vi "Spi Master 128-bit.vi"(0 "spi input":T1, 5 "manual assert chip select":bool, 7 "start strobe":bool, 9 "data to write":bool[](array[boolean]), 11 "MOSI output enable done":bool=TRUE, 13 "spi transfer settings":T2 {"Direction Change Bit" max=64 step=1; "Transfer Length (bits)" min=1 max=64 step=1}) -> (4 "spi output":T3, 8 "read data valid":bool, 10 "read data":bool[](array[boolean]), 14 "ready for input":bool)   [LabVIEW 2015, in "SPI API.lvlib"]
doc: "<b>This VI must be placed in a single-cycle timed loop for guaranteed behavior.</b>\n\nThis VI implements a SPI master that is compliant with both 4-wire (unidirectional input and output data) and 3-wire (bidirectional input/output data) SPI transfers. \n\nPlease see the documentation included with this example for details on how to include this VI into your application.\n\n\"Start strobe\" should be asserted only when \"data to write\" is valid. \"Data to write\" is latched when the start strobe asserts."
uses:
  <userlib>/_NI SPI IP/FPGA/Controllers/Public/Spi Master Outputs.ctl
  <userlib>/_NI SPI IP/FPGA/Controllers/Public/Transfer Settings.ctl
  <userlib>/_NI SPI IP/FPGA/Controllers/Public/Spi Master Inputs.ctl
  Controls/Controller Interface.ctl
  Controls/Master State.ctl
  SPI API.lvlib
  <userlib>/_NI SPI IP/FPGA/Controllers/NI SPI IP FPGA.lvlib
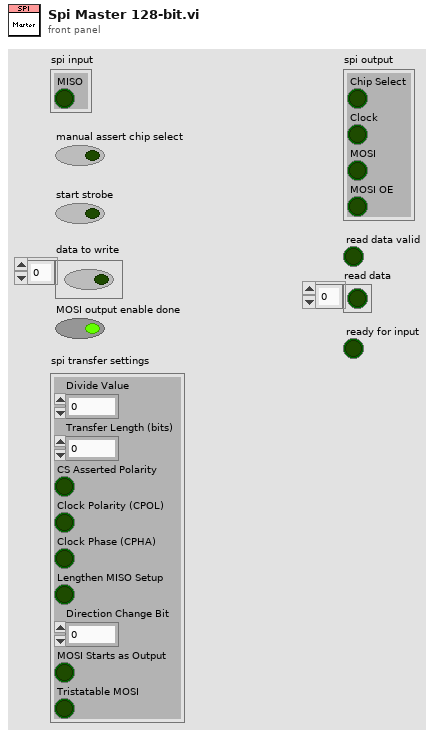
[diagram p1: front panel]
types:
  T1 = typedef "NI SPI IP FPGA.lvlib/Spi Master Inputs.ctl" = cluster{"MISO":bool}
  T2 = typedef "NI SPI IP FPGA.lvlib/Transfer Settings.ctl" = cluster{"Divide Value":u8, "Transfer Length (bits)":u8, "CS Asserted Polarity":bool, "Clock Polarity (CPOL)":bool, "Clock Phase (CPHA)":bool, "Lengthen MISO Setup":bool, "Direction Change Bit":u8, "MOSI Starts as Output":bool, "Tristatable MOSI":bool}
  T3 = typedef "NI SPI IP FPGA.lvlib/Spi Master Outputs.ctl" = cluster{"Chip Select":bool, "Clock":bool, "MOSI":bool, "MOSI OE":bool}
  T4 = typedef "SPI API.lvlib/Master State.ctl" = enum16{"Idle", "Load", "AssertChipSelect", "SendData", "DeassertChipSelect", "Done", "Change MOSI Direction", "WaitForDirChangeDone"}
  T5 = typedef "SPI API.lvlib/Controller Interface.ctl" = cluster{"Load":bool, "Divider Pulse":bool, "Enable Data":bool, "Clear Mosi":bool}
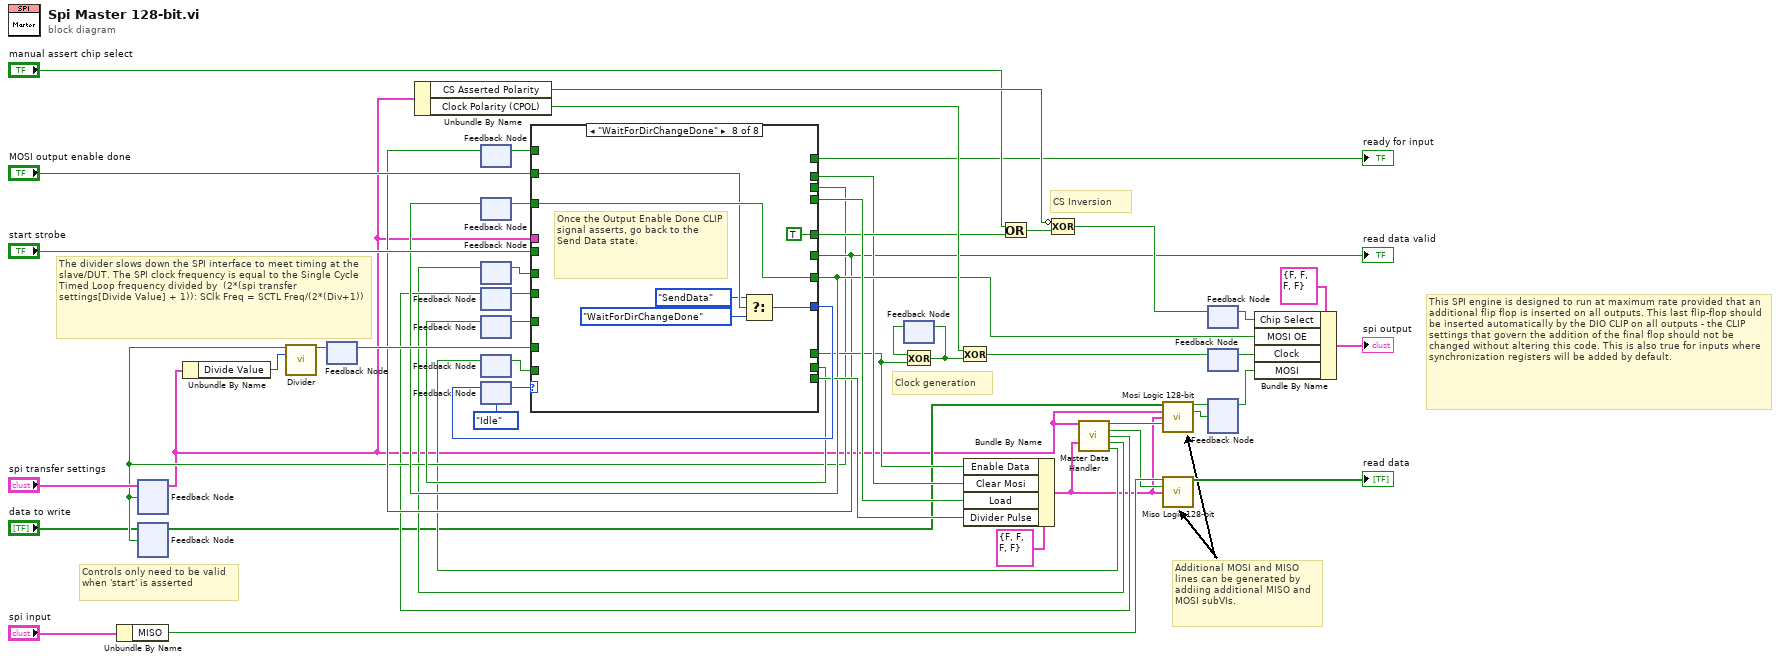
[diagram p0: block diagram]
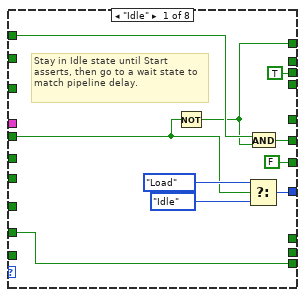
[diagram p2: hidden frame]
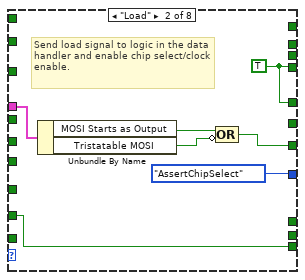
[diagram p3: hidden frame]
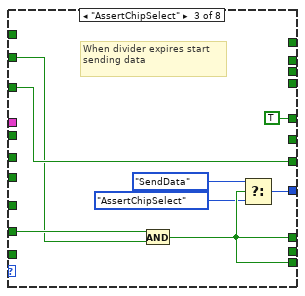
[diagram p4: hidden frame]
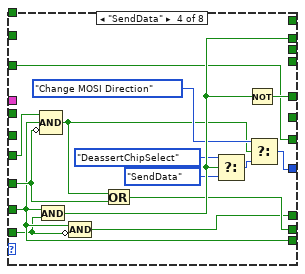
[diagram p5: hidden frame]
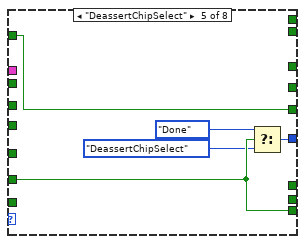
[diagram p6: hidden frame]
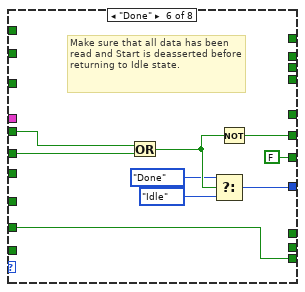
[diagram p7: hidden frame]
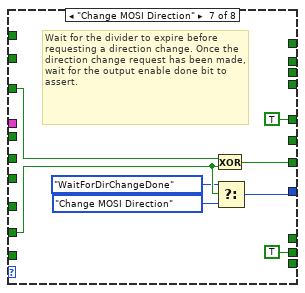
[diagram p8: hidden frame]
diagram:
  # "CS Inversion"
  # "Additional MOSI and MISO lines can be generated by addiing additional MISO and MOSI subVIs."
  # "Controls only need to be valid when 'start' is asserted"
  # "Clock generation"
  # "This SPI engine is designed to run at maximum rate provided that an additional flip flop is inserted on all outputs. This last flip-flop should be inserted automatically by the DIO CLIP on all outputs - the CLIP settings that govern the addition of the final flop should not be changed without altering this code. This is also true for inputs where synchronization registers will be added by default."
  # "The divider slows down the SPI interface to meet timing at the slave/DUT. The SPI clock frequency is equal to the Single Cycle Timed Loop frequency divided by  (2*(spi transfer settings[Divide Value] + 1)): SClk Freq = SCTL Freq/(2*(Div+1))"
  n1 = Unbundle By Name("spi input") -> ("MISO"=w4:bool)
  n2 = feedback #1() -> (w8:T2)  [unwired: 1 in]
  n3 = feedback #2() -> (w9:bool[])  [unwired: 1 in]
  n4 = Unbundle By Name(w8) -> ("Divide Value"=w15:u8)
  n5 = feedback #3() -> (w40:bool)  [unwired: 1 in]
  n6 = Unbundle By Name(w8) -> ("CS Asserted Polarity"=w37:bool, "Clock Polarity (CPOL)"=w49:bool)
  n7 = feedback #4() -> (w19:bool)  [unwired: 1 in]
  n8 = feedback #5() -> (w32:bool)  [unwired: 1 in]
  n9 = feedback #6() -> (w43:bool)  [unwired: 1 in]
  n10 = feedback #7() -> (w33:bool)  [unwired: 1 in]
  n11 = feedback #8() -> (w29:bool)  [unwired: 1 in]
  n12 = feedback #9() -> (w50:bool)  [unwired: 1 in]
  n13 = feedback #10(Master_State."Idle" ("state type")) -> (w52:T4)
  n14 = case shown="\"WaitForDirChangeDone\"" w52 {
    tunnel: [w63 Master_State."AssertChipSelect" ("state type") w78 w90 w98 w107 w114 w120] -> w53
    tunnel: w40 -> [w61 w69 w75 w87 w96 w104 w110 _]
    tunnel: [w58 _ _ _ _ _ _ _] -> w21
    tunnel: "start strobe" -> [w54 _ _ _ _ w106 _ _]
    tunnel: [_ w70 TRUE w93 _ _ TRUE ("Clock") TRUE ("Clock")] -> w36
    tunnel: w50 -> [_ _ _ w86 _ _ _ _]
    tunnel: [_ _ w73 w85 _ _ _ _] -> w22
    tunnel: [_ w70 _ _ _ _ _ _] -> w47
    tunnel: [TRUE ("Clock") _ _ _ _ _ _ _] -> w16
    tunnel: [_ _ _ w92 _ _ _ _] -> w23
    tunnel: w43 -> [_ _ _ _ _ w105 _ _]
    tunnel: w33 -> [_ _ _ w83 _ _ _ _]
    tunnel: [FALSE w65 w76 w84 w97 FALSE w111 w121] -> w24
    tunnel: w32 -> [_ _ w76 w84 w97 _ w112 w121]
    tunnel: [w61 w69 w73 w87 w96 w104 _ _] -> w31
    tunnel: [_ _ _ w88 _ _ TRUE _] -> w30
    tunnel: w29 -> [_ _ _ w89 _ _ _ _]
    tunnel: w8 -> [_ w68 _ _ _ _ _ _]
    tunnel: "MOSI output enable done" -> [_ _ w74 _ _ _ _ w118]
    tunnel: [w60 _ _ _ _ w102 _ _] -> w20
    tunnel: w19 -> [w59 _ _ _ _ _ _ _]
    frame "Idle" {
      # "Stay in Idle state until Start asserts, then go to a wait state to match pipeline delay."
      n15 = Not(x=w54) -> (.not. x?=w58:bool)
      n16 = Select(t=Master_State."Load" ("state type"), s=w54, f=Master_State."Idle" ("state type")) -> (s? t:f=w63:T4)
      n17 = And(x=w59, y=w58) -> (x .and. y?=w60:bool)
    }
    frame "Load" {
      w70 = TRUE ("Clock")
      # "Send load signal to logic in the data handler and enable chip select/clock enable."
      n18 = Unbundle By Name(w68) -> ("MOSI Starts as Output"=w67:bool, "Tristatable MOSI"=w66:bool)
      n19 = Compound Arithmetic op=OR(w67, invert w66) -> (w65:bool)
    }
    frame "AssertChipSelect" {
      # "When divider expires start sending data"
      n20 = And(x=w75, y=w74) -> (x .and. y?=w73:bool)
      n21 = Select(t=Master_State."SendData" ("state type"), s=w73, f=Master_State."AssertChipSelect" ("state type")) -> (s? t:f=w78:T4)
    }
    frame "SendData" {
      n22 = And(x=w87, y=w86) -> (x .and. y?=w92:bool)
      n23 = Compound Arithmetic op=AND(w83, w87, invert w89) -> (w81:bool)
      n24 = Compound Arithmetic op=AND(w87, invert w86) -> (w85:bool)
      n25 = Or(x=w81, y=w89) -> (x .or. y?=w88:bool)
      n26 = Select(t=Master_State."DeassertChipSelect" ("state type"), s=w92, f=Master_State."SendData" ("state type")) -> (s? t:f=w91:T4)
      n27 = Not(x=w92) -> (.not. x?=w93:bool)
      n28 = Select(t=Master_State."Change MOSI Direction" ("state type"), s=w81, f=w91) -> (s? t:f=w90:T4)
    }
    frame "DeassertChipSelect" {
      n29 = Select(t=Master_State."Done" ("state type"), s=w96, f=Master_State."DeassertChipSelect" ("state type")) -> (s? t:f=w98:T4)
    }
    frame "Done" {
      # "Make sure that all data has been read and Start is deasserted before returning to Idle state."
      n30 = Or(x=w106, y=w105) -> (x .or. y?=w103:bool)
      n31 = Select(t=Master_State."Done" ("state type"), s=w103, f=Master_State."Idle" ("state type")) -> (s? t:f=w107:T4)
      n32 = Not(x=w103) -> (.not. x?=w102:bool)
    }
    frame "Change MOSI Direction" {
      # "Wait for the divider to expire before requesting a direction change. Once the direction change request has been made, wait for the output enable done bit to assert."
      n33 = Exclusive Or(1:w110, 2:w112) -> (0:w111:bool)
      n34 = Select(t=Master_State."WaitForDirChangeDone" ("state type"), s=w110, f=Master_State."Change MOSI Direction" ("state type")) -> (s? t:f=w114:T4)
    }
    frame "WaitForDirChangeDone" {
      # "Once the Output Enable Done CLIP signal asserts, go back to the Send Data state."
      n35 = Select(t=Master_State."SendData" ("state type"), s=w118, f=Master_State."WaitForDirChangeDone" ("state type")) -> (s? t:f=w120:T4)
    }
  }
  "ready for input" <- w21
  "read data valid" <- w20
  n36 = feedback-in #1("spi transfer settings", w16) -> ()
  n37 = feedback-in #2("data to write", w16) -> ()
  n38 = call "Divider.vi"("reset"=w16, "divide value"=w15) -> ("count done"=w14:bool)  [unwired: 13 in]
  n39 = feedback-in #3(w14) -> ()
  n40 = feedback-in #4(w20) -> ()
  n41 = feedback-in #5(w24) -> ()
  n42 = feedback-in #8(w30) -> ()
  n43 = feedback-in #10(w53) -> ()
  n44 = feedback #11() -> (w46:bool)  [unwired: 1 in]
  n45 = Exclusive Or(1:w22, 2:w46) -> (0:w34:bool)
  n46 = feedback-in #11(w34) -> ()
  n47 = Exclusive Or(1:w34, 2:w49) -> (0:w48:bool)
  n48 = Bundle By Name(cluster=T5 {"Load"=FALSE, "Divider Pulse"=FALSE, "Enable Data"=FALSE, "Clear Mosi"=FALSE} ("ControllerInterface"), "Enable Data"=w22, "Clear Mosi"=w23, "Load"=w47, "Divider Pulse"=w31) -> (w2:T5)
  n49 = Or(x="manual assert chip select", y=w36) -> (x .or. y?=w27:bool)
  n50 = Compound Arithmetic op=XOR(invert w37, w27) -> (w45:bool)
  n51 = call "Master Data Handler.vi"("transfer settings"=w8, "controller interface"=w2) -> ("shift MOSI"=w7:bool, "sample MISO"=w3:bool, "dir change"=w13:bool, "read pending"=w12:bool, "done"=w11:bool)  [unwired: 9 in]
  n52 = feedback-in #6(w12) -> ()
  n53 = feedback-in #7(w13) -> ()
  n54 = feedback-in #9(w11) -> ()
  n55 = call "Mosi Logic 128-bit.vi"("data to send"=w9, "transfer settings"=w8, "controller interface"=w2, "shift MOSI"=w7) -> ("MOSI"=w6:bool, "MOSI enable"=w5:bool)  [unwired: 10 in]
  n56 = call "Miso Logic 128-bit.vi"("MISO"=w4, "sample MISO"=w3, "controller interface"=w2) -> ("read data"=→"read data":bool[])  [unwired: 12 in]
  n57 = feedback #12() -> (w44:bool)  [unwired: 1 in]
  n58 = feedback-in #12(w45) -> ()
  n59 = feedback #13() -> (w25:bool)  [unwired: 1 in]
  n60 = feedback-in #13(w48) -> ()
  n61 = feedback #14() -> (w26:bool)  [unwired: 1 in]
  n62 = feedback-in #14(w6, w5) -> ()
  n63 = Bundle By Name(cluster=T3 {"Chip Select"=FALSE, "Clock"=FALSE, "MOSI"=FALSE, "MOSI OE"=FALSE} ("SPI.Output"), "Chip Select"=w44, "MOSI OE"=w24, "Clock"=w25, "MOSI"=w26) -> (→"spi output":T3)
